vi "test_ThreeSess_CallGetSession_ReturnsError.vi"(8 "error in":errorcluster) -> (0 "error out":errorcluster, 2 "result":string, 3 "pass":bool)   [LabVIEW 2020, in "MeasurementServerTests.lvlib"]
uses:
  MeasurementServerTests.lvlib
  Runtime/Measurements/Measurement Plugin Session Management V1/Session Reservation/Session Reservation.lvclass
  Runtime/Measurements/Measurement Plugin Session Management V1/Session Reservation/Get Session Info - 1Sess .vi
  Runtime/Measurements/Measurement Plugin Measurement Server/Helpers/Error Strings Global Internal.vi
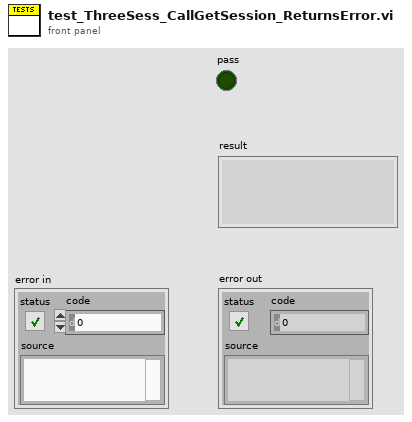
[diagram p1: front panel]
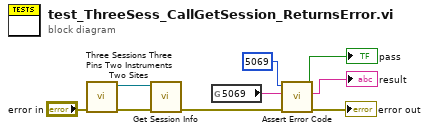
[diagram p0: block diagram]
diagram:
  n1 = call "Three Sessions Three Pins Two Instruments Two Sites.vi"("error in"="error in") -> ("error out"=w2:errorcluster, "session reservation out"=w1:refnum<class "Session Reservation.lvclass">)  [unwired: 8 in, 1 out]
  n2 = call-poly "Get Session Info.vi"("error in"=w2, "session reservation in"=w1) -> ("error out"=w6:errorcluster)  [unwired: 7 in, 2 out]
  n3 = global read "Error Strings Global Internal.vi" "5069"() -> (w7:string)
  n4 = call "Assert Error Code.vi"("error in"=w6, "expected error description"=w7, "expected error code"=5069) -> ("error out"=→"error out":errorcluster, "details"=→"result":string, "error code match?"=→"pass":bool)  [unwired: 6 in]
